vi "Write Keep action_.vi"(8 "error in (no error)":errorcluster, 10 "Keep action?":bool, 11 "AndrewF in":refnum<class "AndrewF.lvclass">) -> (0 "error out":errorcluster, 3 "AndrewF out":refnum<class "AndrewF.lvclass">)   [LabVIEW 2015, in "AndrewF.lvclass"]
uses:
  AndrewF.lvclass
  AndrewF.lvclass/AndrewF.ctl
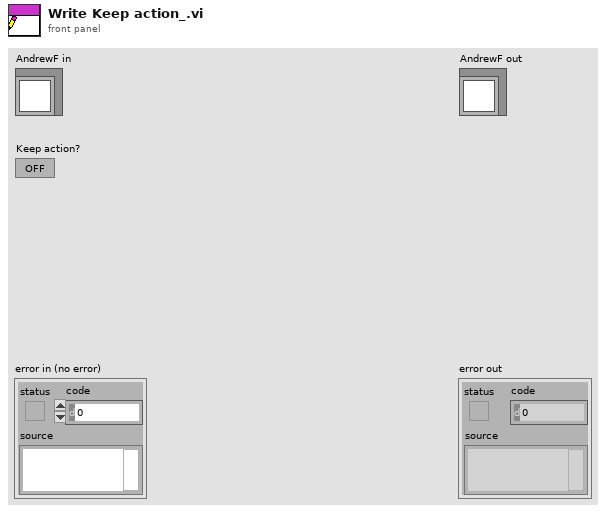
[diagram p1: front panel]
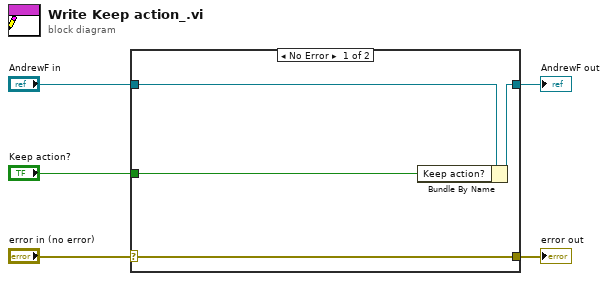
[diagram p0: block diagram]
diagram:
  n1 = case shown="No Error" "error in (no error)" {
    selector: "error in (no error)" -> [w9 w10]
    tunnel: [w9 w10] -> w4
    tunnel: [w7 w11] -> w2
    tunnel: "AndrewF in" -> [w8 w11]
    tunnel: "Keep action?" -> [w6 _]
    frame No Error {
      n2 = Bundle By Name(cluster=w8, "Keep action?"=w6) -> (w7:refnum<class "AndrewF.lvclass">)
    }
    frame Error {
    }
  }
  "error out" <- w4
  "AndrewF out" <- w2
